vi "Simulated.vi"() -> ()   [LabVIEW 2016]
uses:
  <vilib>/rvi/Emulation/niFpgaGetClockAttributes.vi
  <vilib>/rvi/Emulation/niFpgaSctlEmulationGetInTimedLoop.vi
  <vilib>/rvi/Emulation/niFpgaEmulationReportErrorSimple.vi
  <vilib>/rvi/eio/common/nirviEmuTemplateMethod_errors.vi
  <vilib>/rvi/Emulation/niFpgaCriticalErrorInLSC.vi
  <vilib>/eio/EIONode/EIONode.xnode
panel:
  out "Waveform Chart":sgl(graph)
  out "FPGA I/O Out":refnum<k21>
  out "Numeric":fxp<+/-,24,5> format="%.21g"
  in  "stop 2":bool
  out "ON/OFF":bool
  in  "SWITCH":bool
  out "LED 6":bool
  in  "stop":bool
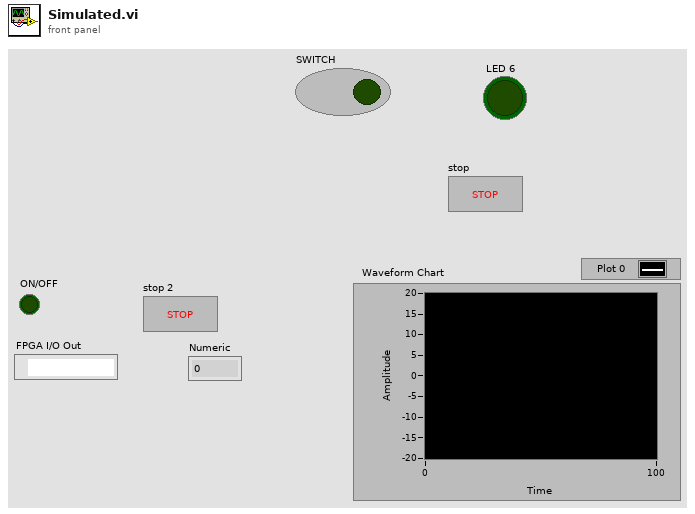
[diagram p1: front panel]
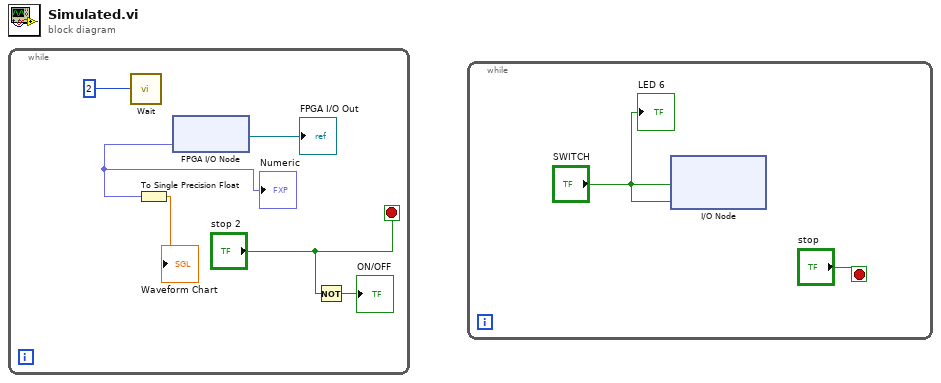
[diagram p0: block diagram]
diagram:
  n1 = while {
    stop <- "stop 2" stop-if-true
    n2 = call "Wait"("Count(mSec)"=u32 2 ("Tick Count(mSec)")) -> ()  [unwired: 1 out]
    n3 = xnode "FPGA I/O Node"() -> ("AI6"=w2:fxp<+/-,24,5>, "FPGA I/O Out"=→"FPGA I/O Out":refnum<k21>)  [unwired: 1 in]
    "Numeric" <- w2
    n4 = To Single Precision Float(number=w2) -> (single precision float=→"Waveform Chart":sgl)
    n5 = Not(x="stop 2") -> (.not. x?=→"ON/OFF":bool)
  }
  n6 = while {
    stop <- "stop" stop-if-true
    n7 = xnode "I/O Node"("FPGA LED"="SWITCH", "DIO9"="SWITCH") -> ()  [unwired: 2 in, 2 out]
    "LED 6" <- "SWITCH"
  }
